vi "Align M + N Waveforms (continuous).vi"(4 "interpolation":bool=TRUE, 6 "FIR filter specifications":T1={"alias rejection (dB)"=120.0, "normalized bandwidth"=0.4536} {"normalized bandwidth" format="%.4f"; "alias rejection (dB)" format="%.2f"}, 7 "reset":bool, 8 "error in (no error)":errorcluster, 9 "interpolation mode":u16(ring)=1 items=["coerce", "linear", "spline", "FIR filter"], 10 "N waveforms in":waveform(dbl)[](array[waveform]), 11 "M waveforms in":waveform(dbl)[](array[waveform])) -> (0 "error out":errorcluster, 2 "N aligned waveforms out":waveform(dbl)[](array[waveform]), 3 "M aligned waveforms out":waveform(dbl)[](array[waveform]))   [LabVIEW 2020, in "NI_MAPro.lvlib"]
doc: "Performs element-wise alignment of waveforms and returns the aligned waveforms. The data types you wire to the waveform inputs determine the polymorphic instance to use."
uses:
  NI_MAPro.lvlib
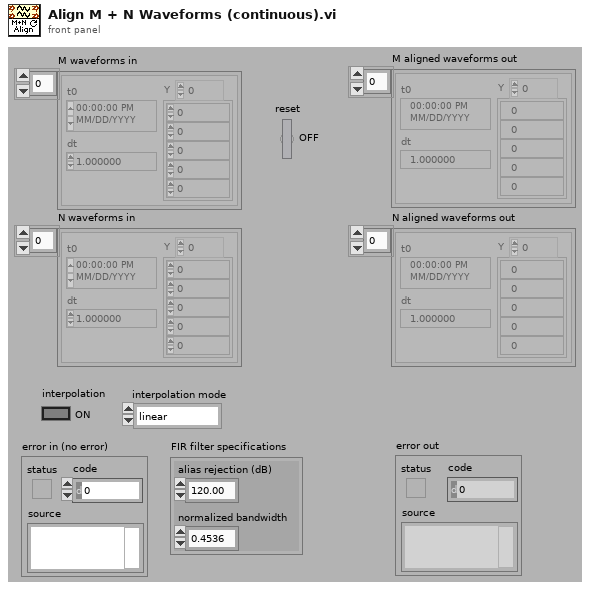
[diagram p1: front panel]
types:
  T1 = cluster{"alias rejection (dB)":dbl, "normalized bandwidth":dbl}
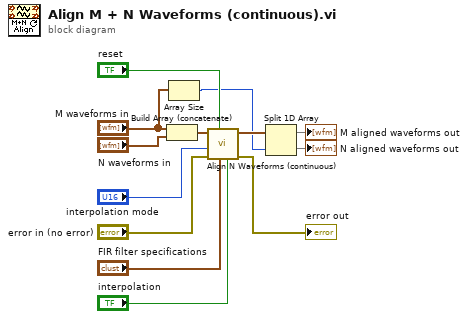
[diagram p0: block diagram]
diagram:
  n1 = Build Array (concatenate)("M waveforms in", "N waveforms in") -> (w9:waveform(dbl)[])
  n2 = Array Size(array="M waveforms in") -> (size(s)=w6:i32)
  n3 = call "Align N Waveforms (continuous).vi"("interpolation"="interpolation", "FIR filter specifications"="FIR filter specifications", "reset"="reset", "error in (no error)"="error in (no error)", "interpolation mode"="interpolation mode", "waveforms in"=w9) -> ("error out"=→"error out":errorcluster, "waveforms out"=w7:waveform(dbl)[])  [unwired: 4 in]
  n4 = Split 1D Array(array=w7, index=w6) -> (first subarray=→"M aligned waveforms out":waveform(dbl)[], second subarray=→"N aligned waveforms out":waveform(dbl)[])
